vi "RN_Inference.vi"(3 "Input Features":dbl[](array[numeric])) -> (1 "Output Probabilities":dbl[](array[numeric]))   [LabVIEW 2025]
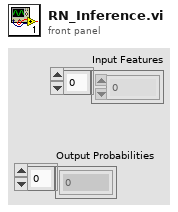
[diagram p1: front panel]
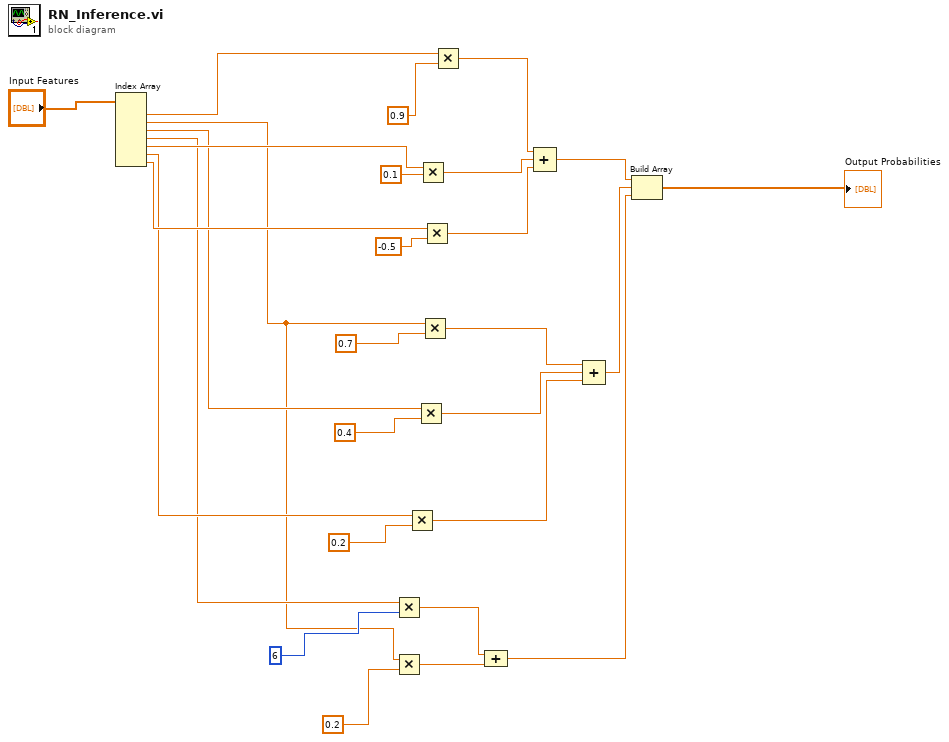
[diagram p0: block diagram]
diagram:
  n1 = Index Array "Index Array"(array="Input Features") -> (element #1=w21:dbl, element #2=w4:dbl, element #3=w12:dbl, element #4=w6:dbl, element #5=w20:dbl, element #6=w11:dbl, element #7=w19:dbl)  [unwired: 7 in]
  n2 = Multiply(x=w6, y=6) -> (x*y=w3:dbl)
  n3 = Multiply(x=w4, y=0.2) -> (x*y=w2:dbl)
  n4 = Multiply(x=w11, y=0.2) -> (x*y=w8:dbl)
  n5 = Multiply(x=w12, y=0.4) -> (x*y=w9:dbl)
  n6 = Multiply(x=w20, y=0.1) -> (x*y=w17:dbl)
  n7 = Multiply(x=w4, y=0.7) -> (x*y=w10:dbl)
  n8 = Multiply(x=w19, y=-0.5) -> (x*y=w16:dbl)
  n9 = Multiply(x=w21, y=0.9) -> (x*y=w18:dbl)
  n10 = Compound Arithmetic op=ADD(w3, w2) -> (w1:dbl)
  n11 = Compound Arithmetic op=ADD(w18, w17, w16) -> (w15:dbl)
  n12 = Compound Arithmetic op=ADD(w10, w9, w8) -> (w7:dbl)
  n13 = Build Array "Build Array"(w15, w7, w1) -> (→"Output Probabilities":dbl[])
